vi "Get I64.vi"(8 "error in (no error)":errorcluster, 9 "Data Type (default value)":i64, 10 "Offset":i32, 11 "JSON":string) -> (0 "error out":errorcluster, 1 "Number":i64, 2 "Offset past match":i32)   [LabVIEW 2024, in "JSONtext.lvlib"]
uses:
  JSONtext.lvlib
  String Subset.vi
  Advance past Number.vi
  Format Error.vi
  Parsing Error in converting to LabVIEW type.vi
  Error Cluster From Error Code.vi
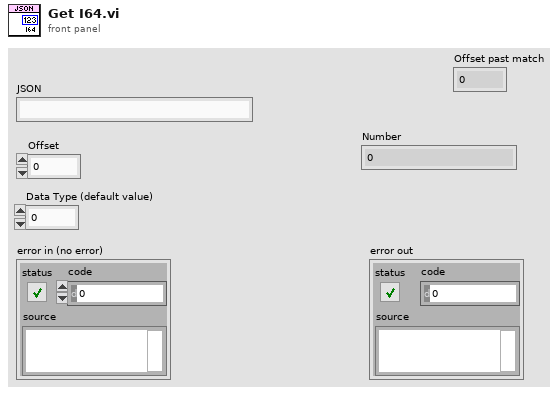
[diagram p1: front panel]
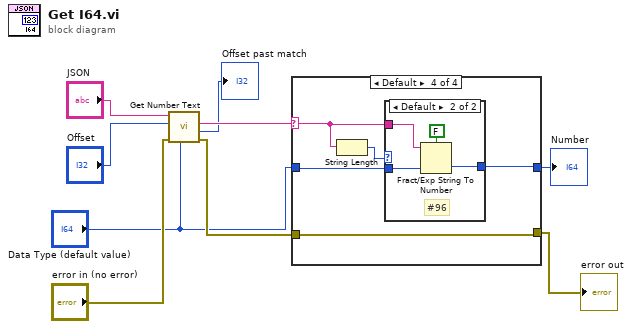
[diagram p0: block diagram]
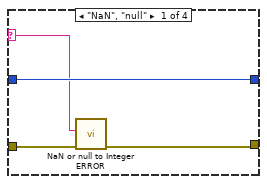
[diagram p2: hidden frame]
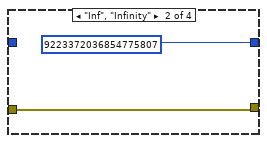
[diagram p3: hidden frame]
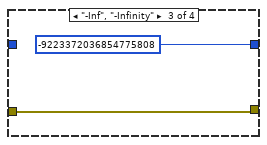
[diagram p4: hidden frame]
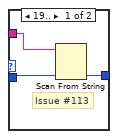
[diagram p5: hidden frame]
diagram:
  n1 = call "Get Number Text.vi"("LV Type"="Data Type (default value)", "error in (no error)"="error in (no error)", "Offset"="Offset", "JSON"="JSON") -> ("error out"=w6:errorcluster, "Offset past match"=→"Offset past match":i32, "Number Text"=w4:string)  [unwired: 4 in, 1 out]
  n2 = case shown="Default" w4 {
    selector: w4 -> [w10 _ _ w20]
    tunnel: [w12 i64 9223372036854775807 ("default value 1") i64 -9223372036854775808 ("default value 1") w18] -> w3
    tunnel: w6 -> [w13 w14 w16 w22]
    tunnel: [w11 w14 w16 w22] -> w5
    tunnel: "Data Type (default value)" -> [w12 _ _ w19]
    frame "NaN", "null" {
      n3 = call "NaN or null to Integer ERROR.vi"("error in (no error)"=w13, "JSON NaN or null"=w10) -> ("error out"=w11:errorcluster)  [unwired: 9 in]
    }
    frame "Inf", "Infinity" {
    }
    frame "-Inf", "-Infinity" {
    }
    frame Default {
      n4 = String Length(string=w20) -> (length=w21:i32)
      n5 = case shown="Default" w21 {
        tunnel: w19 -> [w23 w28]
        tunnel: [w25 w27] -> w18
        tunnel: w20 -> [w24 w26]
        frame 19.. {
          # "Issue #113"
          n6 = Scan From String(input string=w24, default 1=w23) -> (output 1=w25:i64)  [unwired: 3 in, 3 out]
        }
        frame Default {
          # "#96"
          n7 = Fract/Exp String To Number(use system decimal point (T)=FALSE, string=w26, default (0 dbl)=w28) -> (number=w27:i64)  [unwired: 1 in, 1 out]
        }
      }
    }
  }
  "error out" <- w5
  "Number" <- w3
